vi "Adder circuit.vi"() -> ()   [LabVIEW 2025]
panel:
  out "String 2":string="HAlf adder"
  out "carry":bool
  out "sum":bool
  in  "prev carry":bool
  in  "x 2":bool
  in  "y 2":bool
  out "String":string="HAlf adder"
  out "carry":bool
  out "sum":bool
  in  "y":bool
  in  "x":bool
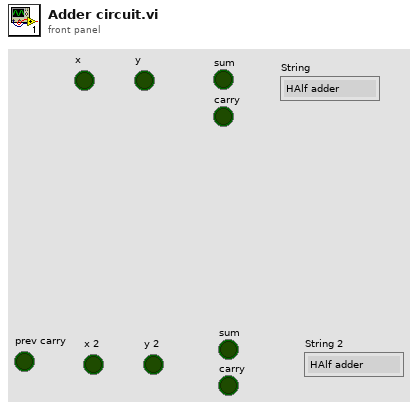
[diagram p1: front panel]
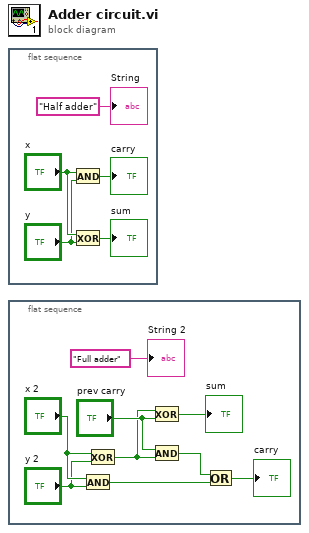
[diagram p0: block diagram]
diagram:
  n1 = flat-sequence {
    frame #0 {
      n2 = And(x="x", y="y") -> (x .and. y?=→"carry":bool)
      n3 = Exclusive Or(1:"y", 2:"x") -> (0:→"sum":bool)
      "String" <- "Half adder"
    }
  }
  n4 = flat-sequence {
    frame #0 {
      n5 = And(x="x 2", y="y 2") -> (x .and. y?=w9:bool)
      n6 = Exclusive Or(1:"y 2", 2:"x 2") -> (0:w11:bool)
      n7 = Exclusive Or(1:"prev carry", 2:w11) -> (0:→"sum":bool)
      n8 = And(x="prev carry", y=w11) -> (x .and. y?=w10:bool)
      n9 = Or(x=w10, y=w9) -> (x .or. y?=→"carry":bool)
      "String 2" <- "Full adder"
    }
  }
